vi "CrossCorrelation PtByPt.vi"(0 "x":dbl format="%0.2f", 1 "sample length x":i32=100, 2 "y":dbl format="%0.2f", 3 "sample length y":i32=100, 4 "initialize":bool) -> (5 "Rxy":dbl[](array[numeric]), 6 "error":i32)   [LabVIEW 2017, in "NI_PtbyPt.lvlib"]
doc: "Computes the cross correlation of <B>x</B> and <B>y</B>."
uses:
  <vilib>/ptbypt/NI_PtbyPt.lvlib
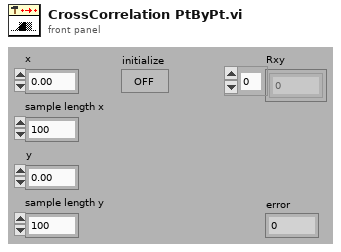
[diagram p1: front panel]
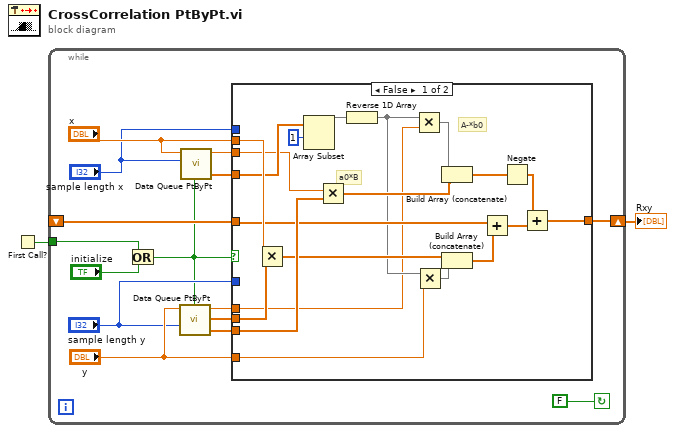
[diagram p0: block diagram]
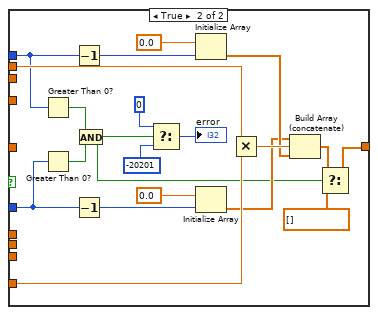
[diagram p2: hidden frame]
diagram:
  n1 = First Call?() -> (First Call?: T/F=w1:bool)
  n2 = while {
    tunnel: w1 -> [w5]
    shift-left: _ -> [w13]
    shift-right: [w17] -> w2
    stop <- FALSE continue-if-true
    n3 = Or(x=w5, y="initialize") -> (x .or. y?=w3:bool)
    n4 = call <vilib>:"Data Queue PtByPt.vi"("initialize"=w3, "sample length"="sample length y", "input data point"="y") -> ("Previous Queue"=w8:dbl[], "Current Queue"=w7:dbl[], "eliminated element"=w9:dbl)  [unwired: 4 in, 2 out]
    n5 = call <vilib>:"Data Queue PtByPt.vi"("initialize"=w3, "sample length"="sample length x", "input data point"="x") -> ("Previous Queue"=w16:dbl[], "eliminated element"=w10:dbl)  [unwired: 4 in, 3 out]
    n6 = case shown="False" w3 {
      tunnel: [w37 w39] -> w17
      tunnel: w16 -> [w20 _]
      tunnel: w8 -> [w36 _]
      tunnel: "y" -> [w35 w56]
      tunnel: "x" -> [w34 w57]
      tunnel: w13 -> [w33 _]
      tunnel: w7 -> [w32 _]
      tunnel: "sample length x" -> [_ w48]
      tunnel: "sample length y" -> [_ w47]
      tunnel: w10 -> [w19 _]
      tunnel: w9 -> [w18 _]
      frame False {
        # "A-*b0"
        # "a0*B"
        n7 = Multiply(x=w34, y=w32) -> (x*y=w27:dbl[])
        n8 = Array Subset(array=w20, index=1 ("Array Index")) -> (w28:dbl[])  [unwired: 1 in]
        n9 = Multiply(x=w19, y=w36) -> (x*y=w29:dbl[])
        n10 = Reverse 1D Array(array=w28) -> (reversed array=w21:dbl[])
        n11 = Multiply(x=w21, y=w18) -> (x*y=w30:dbl[])
        n12 = Multiply(x=w21, y=w35) -> (x*y=w26:dbl[])
        n13 = Build Array (concatenate)(w30, w29) -> (w23:dbl[])
        n14 = Build Array (concatenate)(w27, w26) -> (w25:dbl[])
        n15 = Add(x=w33, y=w25) -> (x+y=w24:dbl[])
        n16 = Negate(x=w23) -> (-x=w22:dbl[])
        n17 = Add(x=w22, y=w24) -> (x+y=w37:dbl[])
      }
      frame True {
        n18 = Greater Than 0?(x=w48) -> (x > 0?=w46:bool)
        n19 = Greater Than 0?(x=w47) -> (x > 0?=w45:bool)
        n20 = Decrement(x=w48) -> (x-1=w54:i32)
        n21 = Decrement(x=w47) -> (x-1=w52:i32)
        n22 = And(x=w46, y=w45) -> (x .and. y?=w44:bool)
        n23 = Select(t=0, s=w44, f=-20201) -> (s? t:f=→"error":i32)
        n24 = Initialize Array(0.0 ("Element Data"), w54) -> (w50:dbl[])
        n25 = Initialize Array(0.0 ("Element Data"), w52) -> (w49:dbl[])
        n26 = Multiply(x=w57, y=w56) -> (x*y=w51:dbl)
        n27 = Build Array (concatenate)(w49, w51, w50) -> (w40:dbl[])
        n28 = Select(t=w40, s=w44, f=dbl[] []) -> (s? t:f=w39:dbl[])
      }
    }
  }
  "Rxy" <- w2
